vi "screen for status.vi"() -> ()   [LabVIEW 2022 SP3]
panel:
  out "?":bool
  out "?":bool
  out "?":bool
  out "?":bool
  out "?":bool
  out "?":bool
  out "?":bool
  # "STATUS"
  # "HEALTH"
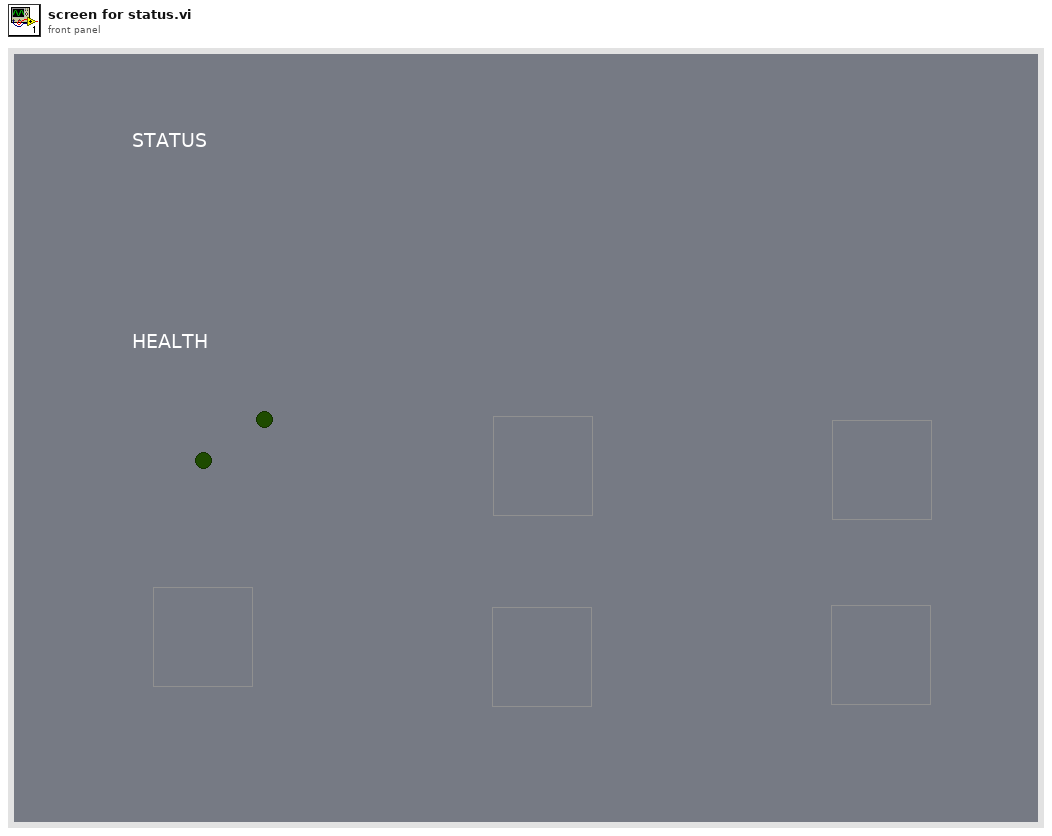
[diagram p1: front panel]
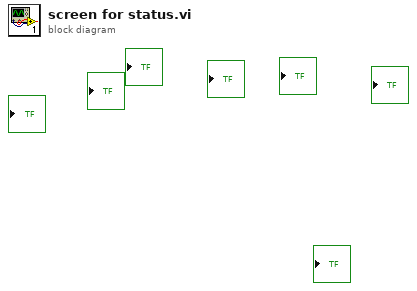
[diagram p0: block diagram]
diagram:
